vi "Mixer.vi"() -> ()   [LabVIEW 2014]
panel:
  in  "?":T1(tab)
  in  "?":bool
  out "Recorded Signal":dynamicdata(graph)
  in  "file path (use dialog)":path
  in  "Sixteenths to Wait":i16(knob) scale=0.0..160.0 scale format="%.1f"
  in  "Eighths":i8(knob) scale=0.0..8.0
  in  "Total Beats":dbl
  in  "BPM":dbl
  in  "Frequency":dbl
  in  "Slide":dbl(slide) scale=0.0..10.0
  in  "file (use dialog)":path
  in  "file (use dialog) 2":path
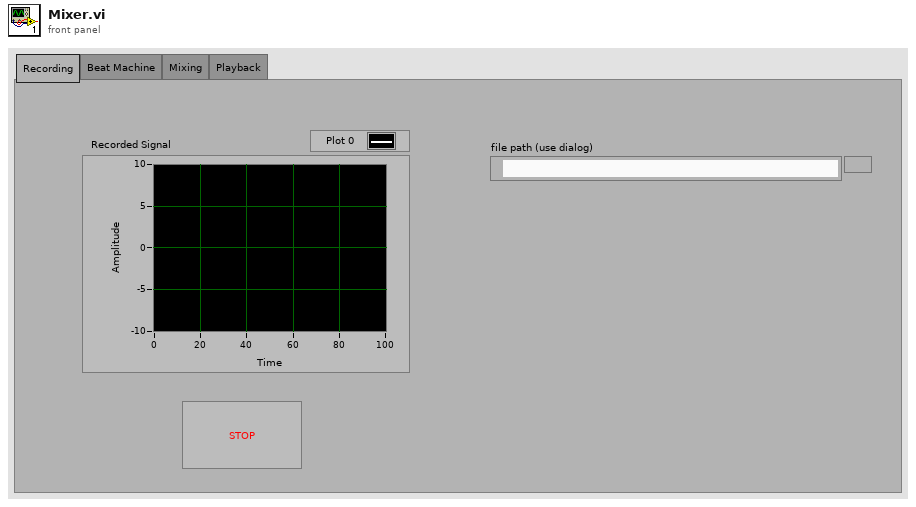
[diagram p1: front panel]
types:
  T1 = enum32{"Recording", "Beat Machine", "Mixing", "Playback"}
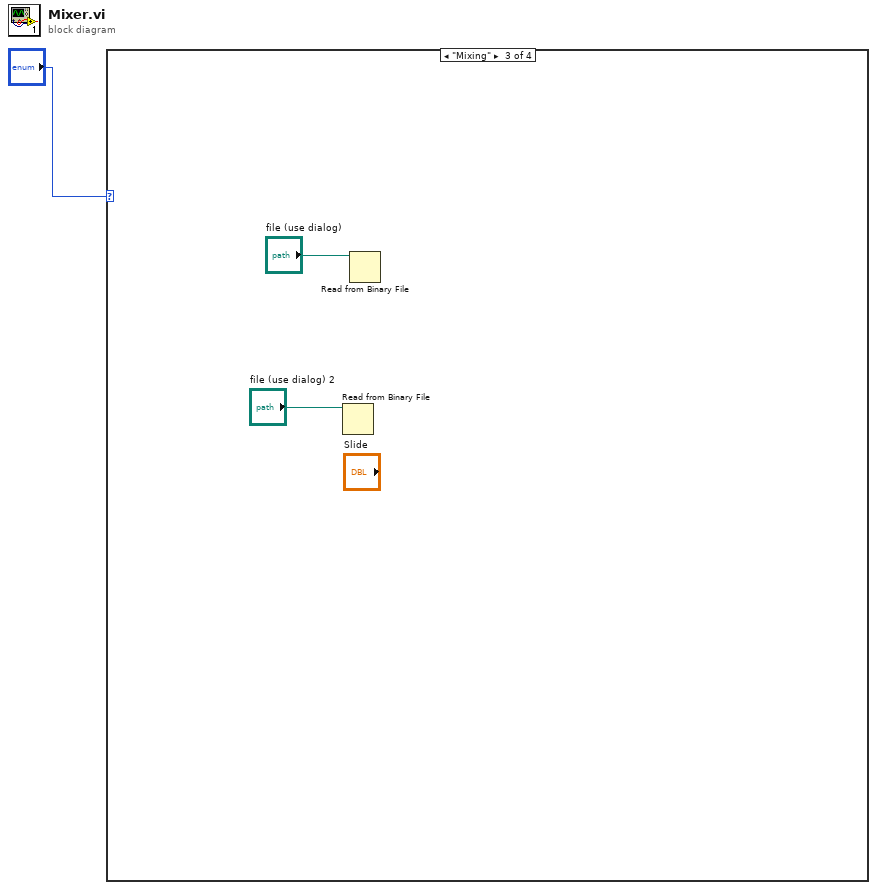
[diagram p0: block diagram]
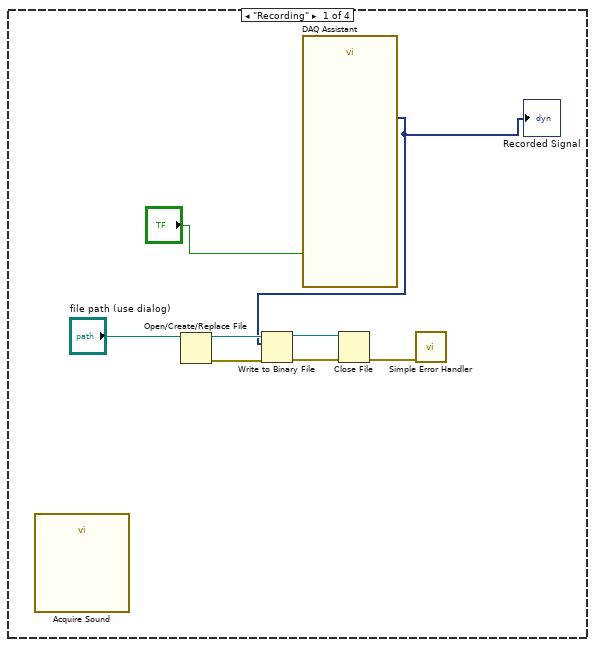
[diagram p2: hidden frame]
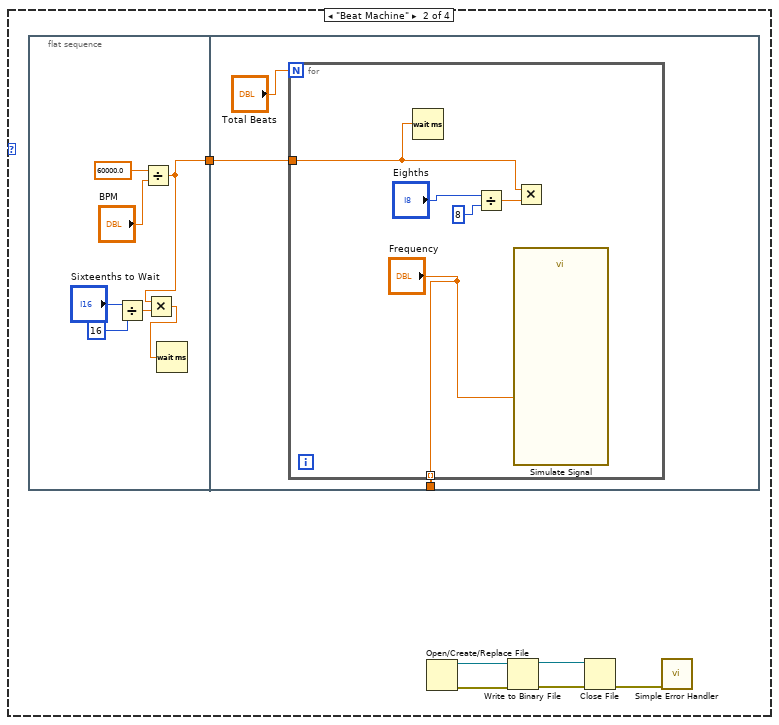
[diagram p3: hidden frame]
diagram:
  n1 = case shown="\"Mixing\"" "?" {
    frame "Recording" {
      n2 = call "Acquire Sound"() -> ()  [unwired: 18 in, 2 out]
      n3 = Open/Create/Replace File(file path (use dialog)="file path (use dialog)") -> (refnum out=w6:refnum<file>, error out=w7:errorcluster)  [unwired: 5 in, 1 out]
      n4 = call "DAQ Assistant"("stop (F)"="?") -> ("data"=w2:dynamicdata)  [unwired: 15 in, 3 out]
      "Recorded Signal" <- w2
      n5 = Write to Binary File(file (use dialog)=w6, data=w2, error in=w7) -> (refnum out=w5:refnum<file>, error out=w4:errorcluster)  [unwired: 3 in, 1 out]
      n6 = Close File(refnum=w5, error in=w4) -> (error out=w3:errorcluster)  [unwired: 1 out]
      n7 = call <vilib>:"Simple Error Handler.vi"("error in (no error)"=w3) -> ()  [unwired: 4 in, 5 out]
    }
    frame "Beat Machine" {
      n8 = flat-sequence {
        tunnel: [w20] -> w18
        tunnel: w18 -> [w27]
        tunnel: [w26] -> w17
        frame #0 {
          n9 = Divide(x="Sixteenths to Wait", y=i16 16) -> (x/y=w23:dbl)
          n10 = Divide(x=60000.0, y="BPM") -> (x/y=w20:dbl)
          n11 = Multiply(x=w20, y=w23) -> (x*y=w19:dbl)
          n12 = Wait (ms)(milliseconds to wait=w19) -> ()  [unwired: 1 out]
        }
        frame #1 {
          n13 = for {
            N: "Total Beats" -> [_]
            tunnel: w27 -> [w30]
            tunnel: ["Frequency"] -> w26 mode=indexing
            n14 = Wait (ms)(milliseconds to wait=w30) -> ()  [unwired: 1 out]
            n15 = Divide(x="Eighths", y=i8 8) -> (x/y=w32:dbl)
            n16 = call "Simulate Signal"("Frequency"="Frequency") -> ()  [unwired: 13 in, 2 out]
            n17 = Multiply(x=w30, y=w32) -> (x*y=w31:dbl)
          }
        }
      }
      n18 = Open/Create/Replace File() -> (file path (use dialog)=w16:path, refnum out=w14:refnum<file>, error out=w15:errorcluster)  [unwired: 5 in, 1 out]
      n19 = Write to Binary File(file (use dialog)=w14, error in=w15) -> (data=w10:cluster{}, refnum out=w13:refnum<file>, error out=w12:errorcluster)  [unwired: 3 in, 1 out]
      n20 = Close File(refnum=w13, error in=w12) -> (error out=w11:errorcluster)  [unwired: 1 out]
      n21 = call <vilib>:"Simple Error Handler.vi"("error in (no error)"=w11) -> ()  [unwired: 4 in, 5 out]
    }
    frame "Mixing" {
      n22 = Read from Binary File(11:"file (use dialog) 2") -> ()  [unwired: 5 in, 4 out]
      n23 = Read from Binary File(11:"file (use dialog)") -> ()  [unwired: 5 in, 4 out]
    }
    frame "Playback" {
    }
  }
